vi "Get Key Names.vi"(5 "Key name/Regex":string, 6 "Context [value]":T1[](array[typedef])=[enum."value"], 7 "Section name/Regex":string, 8 "error in (no error)":errorcluster, 9 "Use Key Regex? [F]":bool, 10 "Use Section Regex? [F]":bool, 11 "Carya Config in":refnum<class "Carya Config.lvclass">) -> (0 "error out":errorcluster, 1 "Key names":string[](array[string]), 2 "Section names":string[](array[string]), 3 "Carya Config out":refnum<class "Carya Config.lvclass">, 4 "Context (concatenated)":string[](array[string]))   [LabVIEW 2013, in "Carya Config.lvclass"]
doc: "Copyright 2018, Carya Automatisering, Wiebe Walstra."
uses:
  Carya Config.lvclass
  CConfig Object/Data.ctl
  CConfig Object/Add Results Query/Add Results Query.lvclass
  CConfig Object/CConfig Object.lvclass
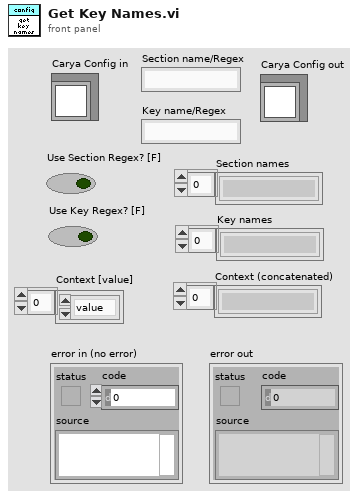
[diagram p1: front panel]
types:
  T1 = typedef "CConfig Object.lvclass/Data.ctl" = enum16{"pre", "name", "middle", "value", "post", "newline", "persistant", "tagged", "type"}
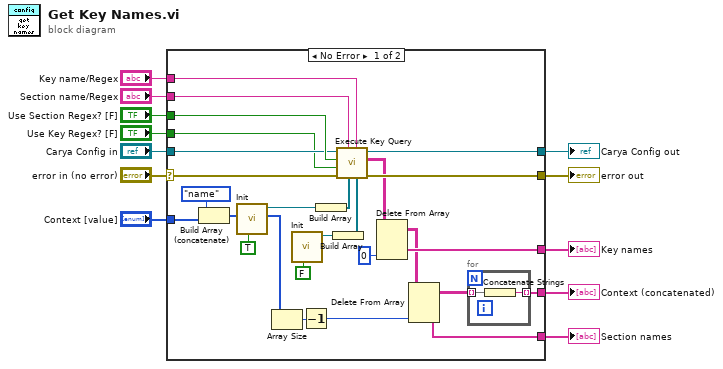
[diagram p0: block diagram]
diagram:
  n1 = case shown="No Error" "error in (no error)" {
    selector: "error in (no error)" -> [w38 w42]
    tunnel: [w33 w42] -> w11
    tunnel: [w32 w41] -> w9
    tunnel: "Carya Config in" -> [w34 w41]
    tunnel: "Section name/Regex" -> [w37 _]
    tunnel: "Use Section Regex? [F]" -> [w36 _]
    tunnel: "Key name/Regex" -> [w28 _]
    tunnel: "Use Key Regex? [F]" -> [w29 _]
    tunnel: [w14 _] -> w3
    tunnel: [w35 _] -> w4
    tunnel: [w31 _] -> w2
    tunnel: "Context [value]" -> [w30 _]
    frame No Error {
      n2 = Build Array (concatenate)(Data."name" ("Data [name]"), w30) -> (w22:T1[])
      n3 = call "Init.vi"("Concatenate\\Build [T, Concatenate]"=TRUE ("Concatenate\\Build [T, Concatenate]"), "Data [name]"=w22) -> ("Find First Query out"=w20:refnum<class "Add Results Query.lvclass">)  [unwired: 8 in, 1 out]
      n4 = Array Size(array=w22) -> (size(s)=w21:i32)
      n5 = call "Init.vi"("Concatenate\\Build [T, Concatenate]"=FALSE ("Concatenate\\Build [T, Concatenate]")) -> ("Find First Query out"=w19:refnum<class "Add Results Query.lvclass">)  [unwired: 9 in, 1 out]
      n6 = Decrement(x=w21) -> (x-1=w15:i32)
      n7 = Build Array(w20) -> (w17:refnum<class "Add Results Query.lvclass">[])
      n8 = Build Array(w19) -> (w18:refnum<class "Add Results Query.lvclass">[])
      n9 = call-dynamic "Execute Key Query.vi"("Section queries"=w18, "Key name"=w28, "Key queries"=w17, "Section name"=w37, "error in (no error)"=w38, "Use Key Regex? [F]"=w29, "Use Section Regex? [F]"=w36, "Carya Config in"=w34) -> ("error out"=w33:errorcluster, "Results"=w24:string[][], "Carya Config out"=w32:refnum<class "Carya Config.lvclass">)  [unwired: 1 in]
      n10 = Delete From Array(array=w24, index (col)=0 ("disabled index (col)")) -> (deleted portion=w35:string[], array with subset deleted=w16:string[][])  [unwired: 2 in]
      n11 = Delete From Array(array=w16, index (col)=w15) -> (deleted portion=w14:string[], array with subset deleted=w13:string[][])  [unwired: 2 in]
      n12 = for {
        tunnel: w13 -> [w40] mode=indexing
        tunnel: [w39] -> w31 mode=indexing
        n13 = Concatenate Strings(w40) -> (w39:string)
      }
    }
    frame Error {
    }
  }
  "error out" <- w11
  "Carya Config out" <- w9
  "Section names" <- w3
  "Key names" <- w4
  "Context (concatenated)" <- w2
